vi "Initailize.vi"(8 "error in (no error)":errorcluster, 9 "zeromq.lvlib:ZeroMQ Context":refnum<class "zmq_context.lvclass">, 10 "Name":string, 11 "Channel Req in":refnum<class "Channel Req.lvclass">) -> (0 "error out":errorcluster, 3 "Channel Req out":refnum<class "Channel Req.lvclass">)   [LabVIEW 2018, in "Channel Req.lvclass"]
uses:
  Channel Req.lvclass
  <vilib>/addons/zeromq/zmq_context.lvclass
  Communication Channel/Communication Channel.lvclass
  Socket/Socket.lvclass
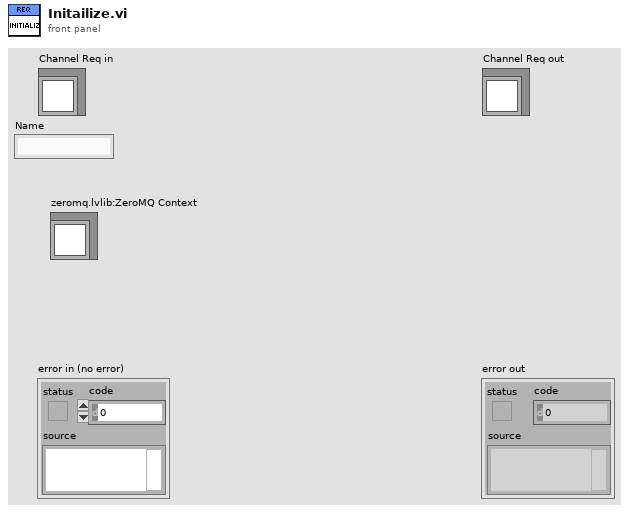
[diagram p1: front panel]
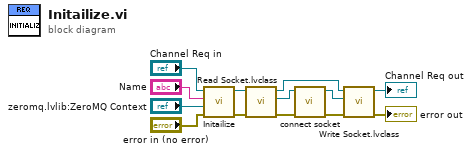
[diagram p0: block diagram]
diagram:
  n1 = call-parent "Initailize.vi"("error in (no error)"="error in (no error)", "zeromq.lvlib:ZeroMQ Context"="zeromq.lvlib:ZeroMQ Context", "Name"="Name", "Communication Channel in"="Channel Req in") -> ("error out"=w5:errorcluster, "Communication Channel out"=w6:refnum<class "Channel Req.lvclass">)  [unwired: 6 in]
  n2 = call-dynamic "Read Socket.lvclass.vi"("error in (no error)"=w5, "Communication Channel in"=w6) -> ("error out"=w4:errorcluster, "Socket.lvclass"=w9:refnum<class "Socket.lvclass">, "Communication Channel out"=w7:refnum<class "Channel Req.lvclass">)  [unwired: 7 in]
  n3 = call "connect socket.vi"("error in (no error)"=w4, "Socket in"=w9) -> ("error out"=w3:errorcluster, "Socket out"=w8:refnum<class "Socket.lvclass">)  [unwired: 8 in]
  n4 = call-dynamic "Write Socket.lvclass.vi"("error in (no error)"=w3, "Socket2.lvclass"=w8, "Communication Channel in"=w7) -> ("error out"=→"error out":errorcluster, "Communication Channel out"=→"Channel Req out":refnum<class "Channel Req.lvclass">)  [unwired: 7 in]
